vi "AndorCreaterErrorCluster.vi"() -> (3 "Array":cluster{i32, string}[](array[cluster]))   [LabVIEW 2018]
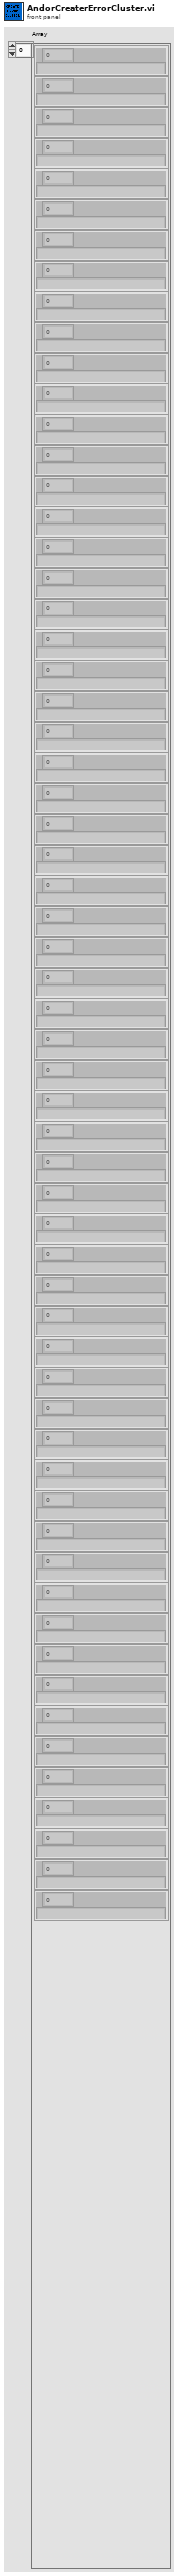
[diagram p1: front panel]
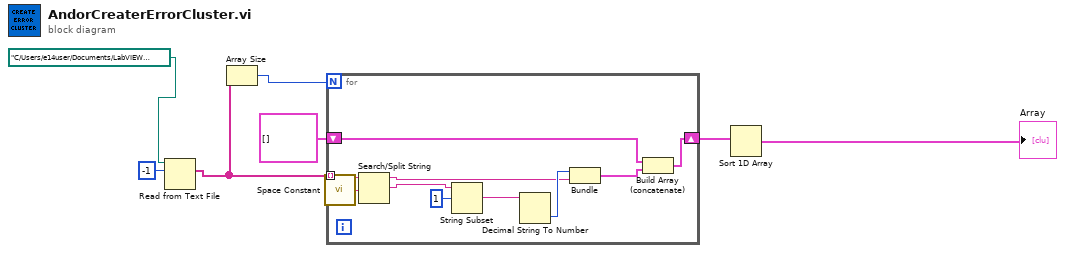
[diagram p0: block diagram]
diagram:
  n1 = Read from Text File(file (use dialog)=path "C:/Users/e14user/Documents/LabVIEW software/GitRepo/lib/ANDOR/CameraErrorCodes.txt", count=-1) -> (text=w4:string[])  [unwired: 2 in, 3 out]
  n2 = Array Size(array=w4) -> (size(s)=w5:i32)
  n3 = for {
    N: w5 -> [_]
    tunnel: w4 -> [w17] mode=indexing
    shift-right: [w10] -> w6
    shift-left: cluster{i32, string}[] [] -> [w11]
    n4 = call <vilib>:"Space Constant.vi"() -> ("String"=w16:string)
    n5 = Search/Split String(string=w17, search string/char (-)=w16) -> (substring before match=w8:string, match + rest of string=w14:string)  [unwired: 1 in, 1 out]
    n6 = String Subset(string=w14, offset (0)=1) -> (substring=w13:string)  [unwired: 1 in]
    n7 = Decimal String To Number(string=w13) -> (number=w9:i32)  [unwired: 2 in, 1 out]
    n8 = Bundle(w9, w8) -> (w12:cluster{i32, string})  [unwired: 1 in]
    n9 = Build Array (concatenate)(w11, w12) -> (w10:cluster{i32, string}[])
  }
  n10 = Sort 1D Array(array=w6) -> (sorted array=→"Array":cluster{i32, string}[])
